vi "输入数据解析.vi"(0 "单个参数补充":dbl, 1 "从板号":dbl=1.0, 2 "主板二维码":string="BNET01", 3 "从板二维码":string="BNET01", 5 "主板引用":refnum<vi>, 7 "从板引用":refnum<vi>, 9 "主板选项":string="三级故障阀值", 11 "枚举":enum16{"主板", "从板"}(ring), 12 "快换":bool caption="快换写入") -> (4 "输出数组":dbl[][](array[numeric]), 6 "数组长度":dbl[](array[numeric]), 8 "循环次数":i32, 10 "命令":u32, 14 "名称":string[](array[string]), 15 "命令序号":u32[](array[numeric]))   [LabVIEW 2013] (continued)
                  disable-tunnel: [w17687 w17691] -> w17683
                  disable-tunnel: w17681 -> [w17686 _]
                  frame Disabled {
                    n6929 = Unbundle By Name(w17686) -> ("电压过高"=w17685:dbl)
                    n6930 = call "输入分辨率计算-EV05.vi"("1字节?"=FALSE, "数值"=w17685, "分辨率"=0.1) -> ("低字节"=w17687:dbl, "高字节1"=w17688:dbl)  [unwired: 2 in, 5 out]
                  }
                  frame Enabled {
                    w17691 = 255 ("高字节1")
                  }
                }
                n6931 = Build Array(w17684, w17683) -> (w17682:i32[])
              }
              frame 1 {
                # "电压过低"
                n6932 = disable-structure shown="启用" {
                  disable-tunnel: [w17699 w17702] -> w17695
                  disable-tunnel: [w17698 w17702] -> w17694
                  disable-tunnel: w17692 -> [w17697 _]
                  frame Disabled {
                    n6933 = Unbundle By Name(w17697) -> ("电压过低"=w17696:dbl)
                    n6934 = call "输入分辨率计算-EV05.vi"("1字节?"=FALSE, "数值"=w17696, "分辨率"=0.1) -> ("低字节"=w17698:dbl, "高字节1"=w17699:dbl)  [unwired: 2 in, 5 out]
                  }
                  frame Enabled {
                    w17702 = 255 ("高字节1")
                  }
                }
                n6935 = Build Array(w17695, w17694) -> (w17693:i32[])
              }
              frame 2 {
                # "电压不均衡"
                n6936 = disable-structure shown="启用" {
                  disable-tunnel: [w17710 w17713] -> w17706
                  disable-tunnel: [w17709 w17713] -> w17705
                  disable-tunnel: w17703 -> [w17708 _]
                  frame Disabled {
                    n6937 = Unbundle By Name(w17708) -> ("电压不均衡(V)"=w17707:dbl)
                    n6938 = call "输入分辨率计算-EV05.vi"("1字节?"=FALSE, "数值"=w17707, "分辨率"=0.1) -> ("低字节"=w17709:dbl, "高字节1"=w17710:dbl)  [unwired: 2 in, 5 out]
                  }
                  frame Enabled {
                    w17713 = 255 ("高字节1")
                  }
                }
                n6939 = Build Array(w17706, w17705) -> (w17704:i32[])
              }
              frame 3 {
                # "温度过高"
                n6940 = disable-structure shown="启用" {
                  disable-tunnel: [w17720 255 ("高字节1")] -> w17716
                  disable-tunnel: w17714 -> [w17718 _]
                  frame Enabled {
                    n6941 = Unbundle By Name(w17718) -> ("温度过高"=w17717:dbl)
                    n6942 = call "输入分辨率计算-EV05.vi"("1字节?"=TRUE, "数值"=w17717, "偏移量"=-40.0, "分辨率"=1.0) -> ("高字节1"=w17720:dbl)  [unwired: 1 in, 6 out]
                  }
                  frame Disabled {
                  }
                }
                n6943 = Build Array(w17716) -> (w17715:dbl[])
              }
              frame 4 {
                # "温度过低"
                n6944 = disable-structure shown="启用" {
                  disable-tunnel: [w17730 255 ("高字节1")] -> w17726
                  disable-tunnel: w17724 -> [w17728 _]
                  frame Disabled {
                    n6945 = Unbundle By Name(w17728) -> ("温度过低"=w17727:dbl)
                    n6946 = call "输入分辨率计算-EV05.vi"("1字节?"=TRUE, "数值"=w17727, "偏移量"=-40.0, "分辨率"=1.0) -> ("高字节1"=w17730:dbl)  [unwired: 1 in, 6 out]
                  }
                  frame Enabled {
                  }
                }
                n6947 = Build Array(w17726) -> (w17725:i32[])
              }
              frame 5 {
                # "温度不均衡"
                n6948 = disable-structure shown="启用" {
                  disable-tunnel: [w17739 255 ("高字节1")] -> w17736
                  disable-tunnel: w17734 -> [w17738 _]
                  frame Disabled {
                    n6949 = Unbundle By Name(w17738) -> ("温度不均衡"=w17737:dbl)
                    n6950 = call "输入分辨率计算-EV05.vi"("1字节?"=TRUE, "数值"=w17737, "分辨率"=1.0) -> ("高字节1"=w17739:dbl)  [unwired: 2 in, 6 out]
                  }
                  frame Enabled {
                  }
                }
                n6951 = Build Array(w17736) -> (w17735:i32[])
              }
              frame 6 {
                # "SOC过低"
                n6952 = disable-structure shown="启用" {
                  disable-tunnel: w17745 -> [w17762 _]
                  disable-tunnel: [w17748 w17765] -> w17744
                  disable-tunnel: [w17747 w17765] -> w17743
                  frame Disabled {
                    n6953 = Unbundle By Name(w17762) -> ("SOC过低"=w17761:dbl)
                    n6954 = call "输入分辨率计算-EV05.vi"("1字节?"=FALSE, "数值"=w17761, "分辨率"=0.1) -> ("低字节"=w17750:dbl, "高字节1"=w17751:dbl)  [unwired: 2 in, 5 out]
                    n6955 = call "二进制解析-8.6.vi"("索引"=4, "数值"=0) -> ("低位子数组"=w17754:i32[])  [unwired: 3 out]
                    n6956 = call "二进制解析-8.6.vi"("索引"=4, "数值"=w17751) -> ("低位子数组"=w17757:i32[])  [unwired: 3 out]
                    n6957 = call "二进制解析-8.6.vi"("索引"=4, "数值"=w17750) -> ("低位子数组"=w17755:i32[], "高位子数组"=w17756:i32[])  [unwired: 2 out]
                    n6958 = Insert Into Array(array=w17757, new element=w17756) -> (w17759:i32[])  [unwired: 1 in]
                    n6959 = Insert Into Array(array=w17755, new element=w17754) -> (w17753:i32[])  [unwired: 1 in]
                    n6960 = call "数值二进制转十进制-8.6.vi"("子数组"=w17753) -> ("十进制数值"=w17748:i32)  [unwired: 4 out]
                    n6961 = call "数值二进制转十进制-8.6.vi"("子数组"=w17759) -> ("十进制数值"=w17747:i32)  [unwired: 4 out]
                  }
                  frame Enabled {
                    w17765 = 255 ("高字节1")
                  }
                }
                n6962 = Build Array(w17743, w17744) -> (w17746:i32[])
              }
            }
            n6963 = Insert Into Array(array=w17677, new element=w17676) -> (w17678:dbl[])  [unwired: 1 in]
          }
          n6964 = Build Array(w17671) -> (w17670:dbl[][])
        }
        frame "温度过高(3)" {
          n6965 = Unbundle By Name(w17770) -> ("三级故障(从板)"=w17771:refnum<vi>)
          n6966 = property class="Clust (严格)"(reference=w17771) -> ("Value"=w17769:T8)  [unwired: 1 in, 2 out]
          n6967 = for {
            N: 7 -> [_]
            tunnel: w17769 -> [w17781]
            shift-right: [w17780] -> w17773
            shift-left: dbl[] [] -> [w17779]
            i -> [w17782]
            n6968 = case shown="3" w17782 {
              tunnel: w17781 -> [w17783 w17794 w17805 w17816 w17826 w17836 w17847]
              tunnel: [w17784 w17795 w17806 w17817 w17827 w17837 w17848] -> w17778
              frame 0, Default {
                # "电压过高"
                n6969 = disable-structure shown="启用" {
                  disable-tunnel: [w17790 w17793] -> w17786
                  disable-tunnel: [w17789 w17793] -> w17785
                  disable-tunnel: w17783 -> [w17788 _]
                  frame Disabled {
                    n6970 = Unbundle By Name(w17788) -> ("电压过高"=w17787:dbl)
                    n6971 = call "输入分辨率计算-EV05.vi"("1字节?"=FALSE, "数值"=w17787, "分辨率"=0.1) -> ("低字节"=w17789:dbl, "高字节1"=w17790:dbl)  [unwired: 2 in, 5 out]
                  }
                  frame Enabled {
                    w17793 = 255 ("高字节1")
                  }
                }
                n6972 = Build Array(w17786, w17785) -> (w17784:i32[])
              }
              frame 1 {
                # "电压过低"
                n6973 = disable-structure shown="启用" {
                  disable-tunnel: [w17801 w17804] -> w17797
                  disable-tunnel: [w17800 w17804] -> w17796
                  disable-tunnel: w17794 -> [w17799 _]
                  frame Disabled {
                    n6974 = Unbundle By Name(w17799) -> ("电压过低"=w17798:dbl)
                    n6975 = call "输入分辨率计算-EV05.vi"("1字节?"=FALSE, "数值"=w17798, "分辨率"=0.1) -> ("低字节"=w17800:dbl, "高字节1"=w17801:dbl)  [unwired: 2 in, 5 out]
                  }
                  frame Enabled {
                    w17804 = 255 ("高字节1")
                  }
                }
                n6976 = Build Array(w17797, w17796) -> (w17795:i32[])
              }
              frame 2 {
                # "电压不均衡"
                n6977 = disable-structure shown="启用" {
                  disable-tunnel: [w17812 w17815] -> w17808
                  disable-tunnel: [w17811 w17815] -> w17807
                  disable-tunnel: w17805 -> [w17810 _]
                  frame Disabled {
                    n6978 = Unbundle By Name(w17810) -> ("电压不均衡(V)"=w17809:dbl)
                    n6979 = call "输入分辨率计算-EV05.vi"("1字节?"=FALSE, "数值"=w17809, "分辨率"=0.1) -> ("低字节"=w17811:dbl, "高字节1"=w17812:dbl)  [unwired: 2 in, 5 out]
                  }
                  frame Enabled {
                    w17815 = 255 ("高字节1")
                  }
                }
                n6980 = Build Array(w17808, w17807) -> (w17806:i32[])
              }
              frame 3 {
                # "温度过高"
                n6981 = disable-structure shown="启用" {
                  disable-tunnel: [w17822 255 ("高字节1")] -> w17818
                  disable-tunnel: w17816 -> [w17820 _]
                  frame Enabled {
                    n6982 = Unbundle By Name(w17820) -> ("温度过高"=w17819:dbl)
                    n6983 = call "输入分辨率计算-EV05.vi"("1字节?"=TRUE, "数值"=w17819, "偏移量"=-40.0, "分辨率"=1.0) -> ("高字节1"=w17822:dbl)  [unwired: 1 in, 6 out]
                  }
                  frame Disabled {
                  }
                }
                n6984 = Build Array(w17818) -> (w17817:dbl[])
              }
              frame 4 {
                # "温度过低"
                n6985 = disable-structure shown="启用" {
                  disable-tunnel: [w17832 255 ("高字节1")] -> w17828
                  disable-tunnel: w17826 -> [w17830 _]
                  frame Disabled {
                    n6986 = Unbundle By Name(w17830) -> ("温度过低"=w17829:dbl)
                    n6987 = call "输入分辨率计算-EV05.vi"("1字节?"=TRUE, "数值"=w17829, "偏移量"=-40.0, "分辨率"=1.0) -> ("高字节1"=w17832:dbl)  [unwired: 1 in, 6 out]
                  }
                  frame Enabled {
                  }
                }
                n6988 = Build Array(w17828) -> (w17827:i32[])
              }
              frame 5 {
                # "温度不均衡"
                n6989 = disable-structure shown="启用" {
                  disable-tunnel: [w17841 255 ("高字节1")] -> w17838
                  disable-tunnel: w17836 -> [w17840 _]
                  frame Disabled {
                    n6990 = Unbundle By Name(w17840) -> ("温度不均衡"=w17839:dbl)
                    n6991 = call "输入分辨率计算-EV05.vi"("1字节?"=TRUE, "数值"=w17839, "分辨率"=1.0) -> ("高字节1"=w17841:dbl)  [unwired: 2 in, 6 out]
                  }
                  frame Enabled {
                  }
                }
                n6992 = Build Array(w17838) -> (w17837:i32[])
              }
              frame 6 {
                # "SOC过低"
                n6993 = disable-structure shown="启用" {
                  disable-tunnel: w17847 -> [w17864 _]
                  disable-tunnel: [w17850 w17867] -> w17846
                  disable-tunnel: [w17849 w17867] -> w17845
                  frame Disabled {
                    n6994 = Unbundle By Name(w17864) -> ("SOC过低"=w17863:dbl)
                    n6995 = call "输入分辨率计算-EV05.vi"("1字节?"=FALSE, "数值"=w17863, "分辨率"=0.1) -> ("低字节"=w17852:dbl, "高字节1"=w17853:dbl)  [unwired: 2 in, 5 out]
                    n6996 = call "二进制解析-8.6.vi"("索引"=4, "数值"=0) -> ("低位子数组"=w17856:i32[])  [unwired: 3 out]
                    n6997 = call "二进制解析-8.6.vi"("索引"=4, "数值"=w17853) -> ("低位子数组"=w17859:i32[])  [unwired: 3 out]
                    n6998 = call "二进制解析-8.6.vi"("索引"=4, "数值"=w17852) -> ("低位子数组"=w17857:i32[], "高位子数组"=w17858:i32[])  [unwired: 2 out]
                    n6999 = Insert Into Array(array=w17859, new element=w17858) -> (w17861:i32[])  [unwired: 1 in]
                    n7000 = Insert Into Array(array=w17857, new element=w17856) -> (w17855:i32[])  [unwired: 1 in]
                    n7001 = call "数值二进制转十进制-8.6.vi"("子数组"=w17855) -> ("十进制数值"=w17850:i32)  [unwired: 4 out]
                    n7002 = call "数值二进制转十进制-8.6.vi"("子数组"=w17861) -> ("十进制数值"=w17849:i32)  [unwired: 4 out]
                  }
                  frame Enabled {
                    w17867 = 255 ("高字节1")
                  }
                }
                n7003 = Build Array(w17845, w17846) -> (w17848:i32[])
              }
            }
            n7004 = Insert Into Array(array=w17779, new element=w17778) -> (w17780:dbl[])  [unwired: 1 in]
          }
          n7005 = Build Array(w17773) -> (w17772:dbl[][])
        }
        frame "温度过低" {
          n7006 = Unbundle By Name(w17872) -> ("一级故障(从板)"=w17873:refnum<vi>)
          n7007 = property class="Clust (严格)"(reference=w17873) -> ("Value"=w17871:T8)  [unwired: 1 in, 2 out]
          n7008 = for {
            N: 7 -> [_]
            tunnel: w17871 -> [w17883]
            shift-right: [w17882] -> w17875
            shift-left: dbl[] [] -> [w17881]
            i -> [w17884]
            n7009 = case shown="4" w17884 {
              tunnel: w17883 -> [w17885 w17896 w17907 w17918 w17928 w17938 w17949]
              tunnel: [w17886 w17897 w17908 w17919 w17929 w17939 w17950] -> w17880
              frame 0, Default {
                # "电压过高"
                n7010 = disable-structure shown="启用" {
                  disable-tunnel: [w17892 w17895] -> w17888
                  disable-tunnel: [w17891 w17895] -> w17887
                  disable-tunnel: w17885 -> [w17890 _]
                  frame Disabled {
                    n7011 = Unbundle By Name(w17890) -> ("电压过高"=w17889:dbl)
                    n7012 = call "输入分辨率计算-EV05.vi"("1字节?"=FALSE, "数值"=w17889, "分辨率"=0.1) -> ("低字节"=w17891:dbl, "高字节1"=w17892:dbl)  [unwired: 2 in, 5 out]
                  }
                  frame Enabled {
                    w17895 = 255 ("高字节1")
                  }
                }
                n7013 = Build Array(w17888, w17887) -> (w17886:i32[])
              }
              frame 1 {
                # "电压过低"
                n7014 = disable-structure shown="启用" {
                  disable-tunnel: [w17903 w17906] -> w17899
                  disable-tunnel: [w17902 w17906] -> w17898
                  disable-tunnel: w17896 -> [w17901 _]
                  frame Disabled {
                    n7015 = Unbundle By Name(w17901) -> ("电压过低"=w17900:dbl)
                    n7016 = call "输入分辨率计算-EV05.vi"("1字节?"=FALSE, "数值"=w17900, "分辨率"=0.1) -> ("低字节"=w17902:dbl, "高字节1"=w17903:dbl)  [unwired: 2 in, 5 out]
                  }
                  frame Enabled {
                    w17906 = 255 ("高字节1")
                  }
                }
                n7017 = Build Array(w17899, w17898) -> (w17897:i32[])
              }
              frame 2 {
                # "电压不均衡"
                n7018 = disable-structure shown="启用" {
                  disable-tunnel: [w17914 w17917] -> w17910
                  disable-tunnel: [w17913 w17917] -> w17909
                  disable-tunnel: w17907 -> [w17912 _]
                  frame Disabled {
                    n7019 = Unbundle By Name(w17912) -> ("电压不均衡(V)"=w17911:dbl)
                    n7020 = call "输入分辨率计算-EV05.vi"("1字节?"=FALSE, "数值"=w17911, "分辨率"=0.1) -> ("低字节"=w17913:dbl, "高字节1"=w17914:dbl)  [unwired: 2 in, 5 out]
                  }
                  frame Enabled {
                    w17917 = 255 ("高字节1")
                  }
                }
                n7021 = Build Array(w17910, w17909) -> (w17908:i32[])
              }
              frame 3 {
                # "温度过高"
                n7022 = disable-structure shown="启用" {
                  disable-tunnel: [w17924 255 ("高字节1")] -> w17920
                  disable-tunnel: w17918 -> [w17922 _]
                  frame Disabled {
                    n7023 = Unbundle By Name(w17922) -> ("温度过高"=w17921:dbl)
                    n7024 = call "输入分辨率计算-EV05.vi"("1字节?"=TRUE, "数值"=w17921, "偏移量"=-40.0, "分辨率"=1.0) -> ("高字节1"=w17924:dbl)  [unwired: 1 in, 6 out]
                  }
                  frame Enabled {
                  }
                }
                n7025 = Build Array(w17920) -> (w17919:i32[])
              }
              frame 4 {
                # "温度过低"
                n7026 = disable-structure shown="启用" {
                  disable-tunnel: [w17934 255 ("高字节1")] -> w17930
                  disable-tunnel: w17928 -> [w17932 _]
                  frame Enabled {
                    n7027 = Unbundle By Name(w17932) -> ("温度过低"=w17931:dbl)
                    n7028 = call "输入分辨率计算-EV05.vi"("1字节?"=TRUE, "数值"=w17931, "偏移量"=-40.0, "分辨率"=1.0) -> ("高字节1"=w17934:dbl)  [unwired: 1 in, 6 out]
                  }
                  frame Disabled {
                  }
                }
                n7029 = Build Array(w17930) -> (w17929:dbl[])
              }
              frame 5 {
                # "温度不均衡"
                n7030 = disable-structure shown="启用" {
                  disable-tunnel: [w17943 255 ("高字节1")] -> w17940
                  disable-tunnel: w17938 -> [w17942 _]
                  frame Disabled {
                    n7031 = Unbundle By Name(w17942) -> ("温度不均衡"=w17941:dbl)
                    n7032 = call "输入分辨率计算-EV05.vi"("1字节?"=TRUE, "数值"=w17941, "分辨率"=1.0) -> ("高字节1"=w17943:dbl)  [unwired: 2 in, 6 out]
                  }
                  frame Enabled {
                  }
                }
                n7033 = Build Array(w17940) -> (w17939:i32[])
              }
              frame 6 {
                # "SOC过低"
                n7034 = disable-structure shown="启用" {
                  disable-tunnel: w17949 -> [w17966 _]
                  disable-tunnel: [w17952 w17969] -> w17948
                  disable-tunnel: [w17951 w17969] -> w17947
                  frame Disabled {
                    n7035 = Unbundle By Name(w17966) -> ("SOC过低"=w17965:dbl)
                    n7036 = call "输入分辨率计算-EV05.vi"("1字节?"=FALSE, "数值"=w17965, "分辨率"=0.1) -> ("低字节"=w17954:dbl, "高字节1"=w17955:dbl)  [unwired: 2 in, 5 out]
                    n7037 = call "二进制解析-8.6.vi"("索引"=4, "数值"=0) -> ("低位子数组"=w17958:i32[])  [unwired: 3 out]
                    n7038 = call "二进制解析-8.6.vi"("索引"=4, "数值"=w17955) -> ("低位子数组"=w17961:i32[])  [unwired: 3 out]
                    n7039 = call "二进制解析-8.6.vi"("索引"=4, "数值"=w17954) -> ("低位子数组"=w17959:i32[], "高位子数组"=w17960:i32[])  [unwired: 2 out]
                    n7040 = Insert Into Array(array=w17961, new element=w17960) -> (w17963:i32[])  [unwired: 1 in]
                    n7041 = Insert Into Array(array=w17959, new element=w17958) -> (w17957:i32[])  [unwired: 1 in]
                    n7042 = call "数值二进制转十进制-8.6.vi"("子数组"=w17957) -> ("十进制数值"=w17952:i32)  [unwired: 4 out]
                    n7043 = call "数值二进制转十进制-8.6.vi"("子数组"=w17963) -> ("十进制数值"=w17951:i32)  [unwired: 4 out]
                  }
                  frame Enabled {
                    w17969 = 255 ("高字节1")
                  }
                }
                n7044 = Build Array(w17947, w17948) -> (w17950:i32[])
              }
            }
            n7045 = Insert Into Array(array=w17881, new element=w17880) -> (w17882:dbl[])  [unwired: 1 in]
          }
          n7046 = Build Array(w17875) -> (w17874:dbl[][])
        }
        frame "温度过低(2)" {
          n7047 = Unbundle By Name(w17974) -> ("二级故障(从板)"=w17975:refnum<vi>)
          n7048 = property class="Clust (严格)"(reference=w17975) -> ("Value"=w17973:T8)  [unwired: 1 in, 2 out]
          n7049 = for {
            N: 7 -> [_]
            tunnel: w17973 -> [w17985]
            shift-right: [w17984] -> w17977
            shift-left: dbl[] [] -> [w17983]
            i -> [w17986]
            n7050 = case shown="4" w17986 {
              tunnel: w17985 -> [w17987 w17998 w18009 w18020 w18030 w18040 w18051]
              tunnel: [w17988 w17999 w18010 w18021 w18031 w18041 w18052] -> w17982
              frame 0, Default {
                # "电压过高"
                n7051 = disable-structure shown="启用" {
                  disable-tunnel: [w17994 w17997] -> w17990
                  disable-tunnel: [w17993 w17997] -> w17989
                  disable-tunnel: w17987 -> [w17992 _]
                  frame Disabled {
                    n7052 = Unbundle By Name(w17992) -> ("电压过高"=w17991:dbl)
                    n7053 = call "输入分辨率计算-EV05.vi"("1字节?"=FALSE, "数值"=w17991, "分辨率"=0.1) -> ("低字节"=w17993:dbl, "高字节1"=w17994:dbl)  [unwired: 2 in, 5 out]
                  }
                  frame Enabled {
                    w17997 = 255 ("高字节1")
                  }
                }
                n7054 = Build Array(w17990, w17989) -> (w17988:i32[])
              }
              frame 1 {
                # "电压过低"
                n7055 = disable-structure shown="启用" {
                  disable-tunnel: [w18005 w18008] -> w18001
                  disable-tunnel: [w18004 w18008] -> w18000
                  disable-tunnel: w17998 -> [w18003 _]
                  frame Disabled {
                    n7056 = Unbundle By Name(w18003) -> ("电压过低"=w18002:dbl)
                    n7057 = call "输入分辨率计算-EV05.vi"("1字节?"=FALSE, "数值"=w18002, "分辨率"=0.1) -> ("低字节"=w18004:dbl, "高字节1"=w18005:dbl)  [unwired: 2 in, 5 out]
                  }
                  frame Enabled {
                    w18008 = 255 ("高字节1")
                  }
                }
                n7058 = Build Array(w18001, w18000) -> (w17999:i32[])
              }
              frame 2 {
                # "电压不均衡"
                n7059 = disable-structure shown="启用" {
                  disable-tunnel: [w18016 w18019] -> w18012
                  disable-tunnel: [w18015 w18019] -> w18011
                  disable-tunnel: w18009 -> [w18014 _]
                  frame Disabled {
                    n7060 = Unbundle By Name(w18014) -> ("电压不均衡(V)"=w18013:dbl)
                    n7061 = call "输入分辨率计算-EV05.vi"("1字节?"=FALSE, "数值"=w18013, "分辨率"=0.1) -> ("低字节"=w18015:dbl, "高字节1"=w18016:dbl)  [unwired: 2 in, 5 out]
                  }
                  frame Enabled {
                    w18019 = 255 ("高字节1")
                  }
                }
                n7062 = Build Array(w18012, w18011) -> (w18010:i32[])
              }
              frame 3 {
                # "温度过高"
                n7063 = disable-structure shown="启用" {
                  disable-tunnel: [w18026 255 ("高字节1")] -> w18022
                  disable-tunnel: w18020 -> [w18024 _]
                  frame Disabled {
                    n7064 = Unbundle By Name(w18024) -> ("温度过高"=w18023:dbl)
                    n7065 = call "输入分辨率计算-EV05.vi"("1字节?"=TRUE, "数值"=w18023, "偏移量"=-40.0, "分辨率"=1.0) -> ("高字节1"=w18026:dbl)  [unwired: 1 in, 6 out]
                  }
                  frame Enabled {
                  }
                }
                n7066 = Build Array(w18022) -> (w18021:i32[])
              }
              frame 4 {
                # "温度过低"
                n7067 = disable-structure shown="启用" {
                  disable-tunnel: [w18036 255 ("高字节1")] -> w18032
                  disable-tunnel: w18030 -> [w18034 _]
                  frame Enabled {
                    n7068 = Unbundle By Name(w18034) -> ("温度过低"=w18033:dbl)
                    n7069 = call "输入分辨率计算-EV05.vi"("1字节?"=TRUE, "数值"=w18033, "偏移量"=-40.0, "分辨率"=1.0) -> ("高字节1"=w18036:dbl)  [unwired: 1 in, 6 out]
                  }
                  frame Disabled {
                  }
                }
                n7070 = Build Array(w18032) -> (w18031:dbl[])
              }
              frame 5 {
                # "温度不均衡"
                n7071 = disable-structure shown="启用" {
                  disable-tunnel: [w18045 255 ("高字节1")] -> w18042
                  disable-tunnel: w18040 -> [w18044 _]
                  frame Disabled {
                    n7072 = Unbundle By Name(w18044) -> ("温度不均衡"=w18043:dbl)
                    n7073 = call "输入分辨率计算-EV05.vi"("1字节?"=TRUE, "数值"=w18043, "分辨率"=1.0) -> ("高字节1"=w18045:dbl)  [unwired: 2 in, 6 out]
                  }
                  frame Enabled {
                  }
                }
                n7074 = Build Array(w18042) -> (w18041:i32[])
              }
              frame 6 {
                # "SOC过低"
                n7075 = disable-structure shown="启用" {
                  disable-tunnel: w18051 -> [w18068 _]
                  disable-tunnel: [w18054 w18071] -> w18050
                  disable-tunnel: [w18053 w18071] -> w18049
                  frame Disabled {
                    n7076 = Unbundle By Name(w18068) -> ("SOC过低"=w18067:dbl)
                    n7077 = call "输入分辨率计算-EV05.vi"("1字节?"=FALSE, "数值"=w18067, "分辨率"=0.1) -> ("低字节"=w18056:dbl, "高字节1"=w18057:dbl)  [unwired: 2 in, 5 out]
                    n7078 = call "二进制解析-8.6.vi"("索引"=4, "数值"=0) -> ("低位子数组"=w18060:i32[])  [unwired: 3 out]
                    n7079 = call "二进制解析-8.6.vi"("索引"=4, "数值"=w18057) -> ("低位子数组"=w18063:i32[])  [unwired: 3 out]
                    n7080 = call "二进制解析-8.6.vi"("索引"=4, "数值"=w18056) -> ("低位子数组"=w18061:i32[], "高位子数组"=w18062:i32[])  [unwired: 2 out]
                    n7081 = Insert Into Array(array=w18063, new element=w18062) -> (w18065:i32[])  [unwired: 1 in]
                    n7082 = Insert Into Array(array=w18061, new element=w18060) -> (w18059:i32[])  [unwired: 1 in]
                    n7083 = call "数值二进制转十进制-8.6.vi"("子数组"=w18059) -> ("十进制数值"=w18054:i32)  [unwired: 4 out]
                    n7084 = call "数值二进制转十进制-8.6.vi"("子数组"=w18065) -> ("十进制数值"=w18053:i32)  [unwired: 4 out]
                  }
                  frame Enabled {
                    w18071 = 255 ("高字节1")
                  }
                }
                n7085 = Build Array(w18049, w18050) -> (w18052:i32[])
              }
            }
            n7086 = Insert Into Array(array=w17983, new element=w17982) -> (w17984:dbl[])  [unwired: 1 in]
          }
          n7087 = Build Array(w17977) -> (w17976:dbl[][])
        }
        frame "温度过低(3)" {
          n7088 = Unbundle By Name(w18076) -> ("三级故障(从板)"=w18077:refnum<vi>)
          n7089 = property class="Clust (严格)"(reference=w18077) -> ("Value"=w18075:T8)  [unwired: 1 in, 2 out]
          n7090 = for {
            N: 7 -> [_]
            tunnel: w18075 -> [w18087]
            shift-right: [w18086] -> w18079
            shift-left: dbl[] [] -> [w18085]
            i -> [w18088]
            n7091 = case shown="4" w18088 {
              tunnel: w18087 -> [w18089 w18100 w18111 w18122 w18132 w18142 w18153]
              tunnel: [w18090 w18101 w18112 w18123 w18133 w18143 w18154] -> w18084
              frame 0, Default {
                # "电压过高"
                n7092 = disable-structure shown="启用" {
                  disable-tunnel: [w18096 w18099] -> w18092
                  disable-tunnel: [w18095 w18099] -> w18091
                  disable-tunnel: w18089 -> [w18094 _]
                  frame Disabled {
                    n7093 = Unbundle By Name(w18094) -> ("电压过高"=w18093:dbl)
                    n7094 = call "输入分辨率计算-EV05.vi"("1字节?"=FALSE, "数值"=w18093, "分辨率"=0.1) -> ("低字节"=w18095:dbl, "高字节1"=w18096:dbl)  [unwired: 2 in, 5 out]
                  }
                  frame Enabled {
                    w18099 = 255 ("高字节1")
                  }
                }
                n7095 = Build Array(w18092, w18091) -> (w18090:i32[])
              }
              frame 1 {
                # "电压过低"
                n7096 = disable-structure shown="启用" {
                  disable-tunnel: [w18107 w18110] -> w18103
                  disable-tunnel: [w18106 w18110] -> w18102
                  disable-tunnel: w18100 -> [w18105 _]
                  frame Disabled {
                    n7097 = Unbundle By Name(w18105) -> ("电压过低"=w18104:dbl)
                    n7098 = call "输入分辨率计算-EV05.vi"("1字节?"=FALSE, "数值"=w18104, "分辨率"=0.1) -> ("低字节"=w18106:dbl, "高字节1"=w18107:dbl)  [unwired: 2 in, 5 out]
                  }
                  frame Enabled {
                    w18110 = 255 ("高字节1")
                  }
                }
                n7099 = Build Array(w18103, w18102) -> (w18101:i32[])
              }
              frame 2 {
                # "电压不均衡"
                n7100 = disable-structure shown="启用" {
                  disable-tunnel: [w18118 w18121] -> w18114
                  disable-tunnel: [w18117 w18121] -> w18113
                  disable-tunnel: w18111 -> [w18116 _]
                  frame Disabled {
                    n7101 = Unbundle By Name(w18116) -> ("电压不均衡(V)"=w18115:dbl)
                    n7102 = call "输入分辨率计算-EV05.vi"("1字节?"=FALSE, "数值"=w18115, "分辨率"=0.1) -> ("低字节"=w18117:dbl, "高字节1"=w18118:dbl)  [unwired: 2 in, 5 out]
                  }
                  frame Enabled {
                    w18121 = 255 ("高字节1")
                  }
                }
                n7103 = Build Array(w18114, w18113) -> (w18112:i32[])
              }
              frame 3 {
                # "温度过高"
                n7104 = disable-structure shown="启用" {
                  disable-tunnel: [w18128 255 ("高字节1")] -> w18124
                  disable-tunnel: w18122 -> [w18126 _]
                  frame Disabled {
                    n7105 = Unbundle By Name(w18126) -> ("温度过高"=w18125:dbl)
                    n7106 = call "输入分辨率计算-EV05.vi"("1字节?"=TRUE, "数值"=w18125, "偏移量"=-40.0, "分辨率"=1.0) -> ("高字节1"=w18128:dbl)  [unwired: 1 in, 6 out]
                  }
                  frame Enabled {
                  }
                }
                n7107 = Build Array(w18124) -> (w18123:i32[])
              }
              frame 4 {
                # "温度过低"
                n7108 = disable-structure shown="启用" {
                  disable-tunnel: [w18138 255 ("高字节1")] -> w18134
                  disable-tunnel: w18132 -> [w18136 _]
                  frame Enabled {
                    n7109 = Unbundle By Name(w18136) -> ("温度过低"=w18135:dbl)
                    n7110 = call "输入分辨率计算-EV05.vi"("1字节?"=TRUE, "数值"=w18135, "偏移量"=-40.0, "分辨率"=1.0) -> ("高字节1"=w18138:dbl)  [unwired: 1 in, 6 out]
                  }
                  frame Disabled {
                  }
                }
                n7111 = Build Array(w18134) -> (w18133:dbl[])
              }
              frame 5 {
                # "温度不均衡"
                n7112 = disable-structure shown="启用" {
                  disable-tunnel: [w18147 255 ("高字节1")] -> w18144
                  disable-tunnel: w18142 -> [w18146 _]
                  frame Disabled {
                    n7113 = Unbundle By Name(w18146) -> ("温度不均衡"=w18145:dbl)
                    n7114 = call "输入分辨率计算-EV05.vi"("1字节?"=TRUE, "数值"=w18145, "分辨率"=1.0) -> ("高字节1"=w18147:dbl)  [unwired: 2 in, 6 out]
                  }
                  frame Enabled {
                  }
                }
                n7115 = Build Array(w18144) -> (w18143:i32[])
              }
              frame 6 {
                # "SOC过低"
                n7116 = disable-structure shown="启用" {
                  disable-tunnel: w18153 -> [w18170 _]
                  disable-tunnel: [w18156 w18173] -> w18152
                  disable-tunnel: [w18155 w18173] -> w18151
                  frame Disabled {
                    n7117 = Unbundle By Name(w18170) -> ("SOC过低"=w18169:dbl)
                    n7118 = call "输入分辨率计算-EV05.vi"("1字节?"=FALSE, "数值"=w18169, "分辨率"=0.1) -> ("低字节"=w18158:dbl, "高字节1"=w18159:dbl)  [unwired: 2 in, 5 out]
                    n7119 = call "二进制解析-8.6.vi"("索引"=4, "数值"=0) -> ("低位子数组"=w18162:i32[])  [unwired: 3 out]
                    n7120 = call "二进制解析-8.6.vi"("索引"=4, "数值"=w18159) -> ("低位子数组"=w18165:i32[])  [unwired: 3 out]
                    n7121 = call "二进制解析-8.6.vi"("索引"=4, "数值"=w18158) -> ("低位子数组"=w18163:i32[], "高位子数组"=w18164:i32[])  [unwired: 2 out]
                    n7122 = Insert Into Array(array=w18165, new element=w18164) -> (w18167:i32[])  [unwired: 1 in]
                    n7123 = Insert Into Array(array=w18163, new element=w18162) -> (w18161:i32[])  [unwired: 1 in]
                    n7124 = call "数值二进制转十进制-8.6.vi"("子数组"=w18161) -> ("十进制数值"=w18156:i32)  [unwired: 4 out]
                    n7125 = call "数值二进制转十进制-8.6.vi"("子数组"=w18167) -> ("十进制数值"=w18155:i32)  [unwired: 4 out]
                  }
                  frame Enabled {
                    w18173 = 255 ("高字节1")
                  }
                }
                n7126 = Build Array(w18151, w18152) -> (w18154:i32[])
              }
            }
            n7127 = Insert Into Array(array=w18085, new element=w18084) -> (w18086:dbl[])  [unwired: 1 in]
          }
          n7128 = Build Array(w18079) -> (w18078:dbl[][])
        }
        frame "温度不均衡" {
          n7129 = Unbundle By Name(w18178) -> ("一级故障(从板)"=w18179:refnum<vi>)
          n7130 = property class="Clust (严格)"(reference=w18179) -> ("Value"=w18177:T8)  [unwired: 1 in, 2 out]
          n7131 = for {
            N: 7 -> [_]
            tunnel: w18177 -> [w18189]
            shift-right: [w18188] -> w18181
            shift-left: dbl[] [] -> [w18187]
            i -> [w18190]
            n7132 = case shown="5" w18190 {
              tunnel: w18189 -> [w18191 w18202 w18213 w18224 w18234 w18244 w18255]
              tunnel: [w18192 w18203 w18214 w18225 w18235 w18245 w18256] -> w18186
              frame 0, Default {
                # "电压过高"
                n7133 = disable-structure shown="启用" {
                  disable-tunnel: [w18198 w18201] -> w18194
                  disable-tunnel: [w18197 w18201] -> w18193
                  disable-tunnel: w18191 -> [w18196 _]
                  frame Disabled {
                    n7134 = Unbundle By Name(w18196) -> ("电压过高"=w18195:dbl)
                    n7135 = call "输入分辨率计算-EV05.vi"("1字节?"=FALSE, "数值"=w18195, "分辨率"=0.1) -> ("低字节"=w18197:dbl, "高字节1"=w18198:dbl)  [unwired: 2 in, 5 out]
                  }
                  frame Enabled {
                    w18201 = 255 ("高字节1")
                  }
                }
                n7136 = Build Array(w18194, w18193) -> (w18192:i32[])
              }
              frame 1 {
                # "电压过低"
                n7137 = disable-structure shown="启用" {
                  disable-tunnel: [w18209 w18212] -> w18205
                  disable-tunnel: [w18208 w18212] -> w18204
                  disable-tunnel: w18202 -> [w18207 _]
                  frame Disabled {
                    n7138 = Unbundle By Name(w18207) -> ("电压过低"=w18206:dbl)
                    n7139 = call "输入分辨率计算-EV05.vi"("1字节?"=FALSE, "数值"=w18206, "分辨率"=0.1) -> ("低字节"=w18208:dbl, "高字节1"=w18209:dbl)  [unwired: 2 in, 5 out]
                  }
                  frame Enabled {
                    w18212 = 255 ("高字节1")
                  }
                }
                n7140 = Build Array(w18205, w18204) -> (w18203:i32[])
              }
              frame 2 {
                # "电压不均衡"
                n7141 = disable-structure shown="启用" {
                  disable-tunnel: [w18220 w18223] -> w18216
                  disable-tunnel: [w18219 w18223] -> w18215
                  disable-tunnel: w18213 -> [w18218 _]
                  frame Disabled {
                    n7142 = Unbundle By Name(w18218) -> ("电压不均衡(V)"=w18217:dbl)
                    n7143 = call "输入分辨率计算-EV05.vi"("1字节?"=FALSE, "数值"=w18217, "分辨率"=0.1) -> ("低字节"=w18219:dbl, "高字节1"=w18220:dbl)  [unwired: 2 in, 5 out]
                  }
                  frame Enabled {
                    w18223 = 255 ("高字节1")
                  }
                }
                n7144 = Build Array(w18216, w18215) -> (w18214:i32[])
              }
              frame 3 {
                # "温度过高"
                n7145 = disable-structure shown="启用" {
                  disable-tunnel: [w18230 255 ("高字节1")] -> w18226
                  disable-tunnel: w18224 -> [w18228 _]
                  frame Disabled {
                    n7146 = Unbundle By Name(w18228) -> ("温度过高"=w18227:dbl)
                    n7147 = call "输入分辨率计算-EV05.vi"("1字节?"=TRUE, "数值"=w18227, "偏移量"=-40.0, "分辨率"=1.0) -> ("高字节1"=w18230:dbl)  [unwired: 1 in, 6 out]
                  }
                  frame Enabled {
                  }
                }
                n7148 = Build Array(w18226) -> (w18225:i32[])
              }
              frame 4 {
                # "温度过低"
                n7149 = disable-structure shown="启用" {
                  disable-tunnel: [w18240 255 ("高字节1")] -> w18236
                  disable-tunnel: w18234 -> [w18238 _]
                  frame Disabled {
                    n7150 = Unbundle By Name(w18238) -> ("温度过低"=w18237:dbl)
                    n7151 = call "输入分辨率计算-EV05.vi"("1字节?"=TRUE, "数值"=w18237, "偏移量"=-40.0, "分辨率"=1.0) -> ("高字节1"=w18240:dbl)  [unwired: 1 in, 6 out]
                  }
                  frame Enabled {
                  }
                }
                n7152 = Build Array(w18236) -> (w18235:i32[])
              }
              frame 5 {
                # "温度不均衡"
                n7153 = disable-structure shown="启用" {
                  disable-tunnel: [w18249 255 ("高字节1")] -> w18246
                  disable-tunnel: w18244 -> [w18248 _]
                  frame Enabled {
                    n7154 = Unbundle By Name(w18248) -> ("温度不均衡"=w18247:dbl)
                    n7155 = call "输入分辨率计算-EV05.vi"("1字节?"=TRUE, "数值"=w18247, "分辨率"=1.0) -> ("高字节1"=w18249:dbl)  [unwired: 2 in, 6 out]
                  }
                  frame Disabled {
                  }
                }
                n7156 = Build Array(w18246) -> (w18245:dbl[])
              }
              frame 6 {
                # "SOC过低"
                n7157 = disable-structure shown="启用" {
                  disable-tunnel: w18255 -> [w18272 _]
                  disable-tunnel: [w18258 w18275] -> w18254
                  disable-tunnel: [w18257 w18275] -> w18253
                  frame Disabled {
                    n7158 = Unbundle By Name(w18272) -> ("SOC过低"=w18271:dbl)
                    n7159 = call "输入分辨率计算-EV05.vi"("1字节?"=FALSE, "数值"=w18271, "分辨率"=0.1) -> ("低字节"=w18260:dbl, "高字节1"=w18261:dbl)  [unwired: 2 in, 5 out]
                    n7160 = call "二进制解析-8.6.vi"("索引"=4, "数值"=0) -> ("低位子数组"=w18264:i32[])  [unwired: 3 out]
                    n7161 = call "二进制解析-8.6.vi"("索引"=4, "数值"=w18261) -> ("低位子数组"=w18267:i32[])  [unwired: 3 out]
                    n7162 = call "二进制解析-8.6.vi"("索引"=4, "数值"=w18260) -> ("低位子数组"=w18265:i32[], "高位子数组"=w18266:i32[])  [unwired: 2 out]
                    n7163 = Insert Into Array(array=w18267, new element=w18266) -> (w18269:i32[])  [unwired: 1 in]
                    n7164 = Insert Into Array(array=w18265, new element=w18264) -> (w18263:i32[])  [unwired: 1 in]
                    n7165 = call "数值二进制转十进制-8.6.vi"("子数组"=w18263) -> ("十进制数值"=w18258:i32)  [unwired: 4 out]
                    n7166 = call "数值二进制转十进制-8.6.vi"("子数组"=w18269) -> ("十进制数值"=w18257:i32)  [unwired: 4 out]
                  }
                  frame Enabled {
                    w18275 = 255 ("高字节1")
                  }
                }
                n7167 = Build Array(w18253, w18254) -> (w18256:i32[])
              }
            }
            n7168 = Insert Into Array(array=w18187, new element=w18186) -> (w18188:dbl[])  [unwired: 1 in]
          }
          n7169 = Build Array(w18181) -> (w18180:dbl[][])
        }
        frame "温度不均衡(2)" {
          n7170 = Unbundle By Name(w18280) -> ("二级故障(从板)"=w18281:refnum<vi>)
          n7171 = property class="Clust (严格)"(reference=w18281) -> ("Value"=w18279:T8)  [unwired: 1 in, 2 out]
          n7172 = for {
            N: 7 -> [_]
            tunnel: w18279 -> [w18291]
            shift-right: [w18290] -> w18283
            shift-left: dbl[] [] -> [w18289]
            i -> [w18292]
            n7173 = case shown="5" w18292 {
              tunnel: w18291 -> [w18293 w18304 w18315 w18326 w18336 w18346 w18357]
              tunnel: [w18294 w18305 w18316 w18327 w18337 w18347 w18358] -> w18288
              frame 0, Default {
                # "电压过高"
                n7174 = disable-structure shown="启用" {
                  disable-tunnel: [w18300 w18303] -> w18296
                  disable-tunnel: [w18299 w18303] -> w18295
                  disable-tunnel: w18293 -> [w18298 _]
                  frame Disabled {
                    n7175 = Unbundle By Name(w18298) -> ("电压过高"=w18297:dbl)
                    n7176 = call "输入分辨率计算-EV05.vi"("1字节?"=FALSE, "数值"=w18297, "分辨率"=0.1) -> ("低字节"=w18299:dbl, "高字节1"=w18300:dbl)  [unwired: 2 in, 5 out]
                  }
                  frame Enabled {
                    w18303 = 255 ("高字节1")
                  }
                }
                n7177 = Build Array(w18296, w18295) -> (w18294:i32[])
              }
              frame 1 {
                # "电压过低"
                n7178 = disable-structure shown="启用" {
                  disable-tunnel: [w18311 w18314] -> w18307
                  disable-tunnel: [w18310 w18314] -> w18306
                  disable-tunnel: w18304 -> [w18309 _]
                  frame Disabled {
                    n7179 = Unbundle By Name(w18309) -> ("电压过低"=w18308:dbl)
                    n7180 = call "输入分辨率计算-EV05.vi"("1字节?"=FALSE, "数值"=w18308, "分辨率"=0.1) -> ("低字节"=w18310:dbl, "高字节1"=w18311:dbl)  [unwired: 2 in, 5 out]
                  }
                  frame Enabled {
                    w18314 = 255 ("高字节1")
                  }
                }
                n7181 = Build Array(w18307, w18306) -> (w18305:i32[])
              }
              frame 2 {
                # "电压不均衡"
                n7182 = disable-structure shown="启用" {
                  disable-tunnel: [w18322 w18325] -> w18318
                  disable-tunnel: [w18321 w18325] -> w18317
                  disable-tunnel: w18315 -> [w18320 _]
                  frame Disabled {
                    n7183 = Unbundle By Name(w18320) -> ("电压不均衡(V)"=w18319:dbl)
                    n7184 = call "输入分辨率计算-EV05.vi"("1字节?"=FALSE, "数值"=w18319, "分辨率"=0.1) -> ("低字节"=w18321:dbl, "高字节1"=w18322:dbl)  [unwired: 2 in, 5 out]
                  }
                  frame Enabled {
                    w18325 = 255 ("高字节1")
                  }
                }
                n7185 = Build Array(w18318, w18317) -> (w18316:i32[])
              }
              frame 3 {
                # "温度过高"
                n7186 = disable-structure shown="启用" {
                  disable-tunnel: [w18332 255 ("高字节1")] -> w18328
                  disable-tunnel: w18326 -> [w18330 _]
                  frame Disabled {
                    n7187 = Unbundle By Name(w18330) -> ("温度过高"=w18329:dbl)
                    n7188 = call "输入分辨率计算-EV05.vi"("1字节?"=TRUE, "数值"=w18329, "偏移量"=-40.0, "分辨率"=1.0) -> ("高字节1"=w18332:dbl)  [unwired: 1 in, 6 out]
                  }
                  frame Enabled {
                  }
                }
                n7189 = Build Array(w18328) -> (w18327:i32[])
              }
              frame 4 {
                # "温度过低"
                n7190 = disable-structure shown="启用" {
                  disable-tunnel: [w18342 255 ("高字节1")] -> w18338
                  disable-tunnel: w18336 -> [w18340 _]
                  frame Disabled {
                    n7191 = Unbundle By Name(w18340) -> ("温度过低"=w18339:dbl)
                    n7192 = call "输入分辨率计算-EV05.vi"("1字节?"=TRUE, "数值"=w18339, "偏移量"=-40.0, "分辨率"=1.0) -> ("高字节1"=w18342:dbl)  [unwired: 1 in, 6 out]
                  }
                  frame Enabled {
                  }
                }
                n7193 = Build Array(w18338) -> (w18337:i32[])
              }
              frame 5 {
                # "温度不均衡"
                n7194 = disable-structure shown="启用" {
                  disable-tunnel: [w18351 255 ("高字节1")] -> w18348
                  disable-tunnel: w18346 -> [w18350 _]
                  frame Enabled {
                    n7195 = Unbundle By Name(w18350) -> ("温度不均衡"=w18349:dbl)
                    n7196 = call "输入分辨率计算-EV05.vi"("1字节?"=TRUE, "数值"=w18349, "分辨率"=1.0) -> ("高字节1"=w18351:dbl)  [unwired: 2 in, 6 out]
                  }
                  frame Disabled {
                  }
                }
                n7197 = Build Array(w18348) -> (w18347:dbl[])
              }
              frame 6 {
                # "SOC过低"
                n7198 = disable-structure shown="启用" {
                  disable-tunnel: w18357 -> [w18374 _]
                  disable-tunnel: [w18360 w18377] -> w18356
                  disable-tunnel: [w18359 w18377] -> w18355
                  frame Disabled {
                    n7199 = Unbundle By Name(w18374) -> ("SOC过低"=w18373:dbl)
                    n7200 = call "输入分辨率计算-EV05.vi"("1字节?"=FALSE, "数值"=w18373, "分辨率"=0.1) -> ("低字节"=w18362:dbl, "高字节1"=w18363:dbl)  [unwired: 2 in, 5 out]
                    n7201 = call "二进制解析-8.6.vi"("索引"=4, "数值"=0) -> ("低位子数组"=w18366:i32[])  [unwired: 3 out]
                    n7202 = call "二进制解析-8.6.vi"("索引"=4, "数值"=w18363) -> ("低位子数组"=w18369:i32[])  [unwired: 3 out]
                    n7203 = call "二进制解析-8.6.vi"("索引"=4, "数值"=w18362) -> ("低位子数组"=w18367:i32[], "高位子数组"=w18368:i32[])  [unwired: 2 out]
                    n7204 = Insert Into Array(array=w18369, new element=w18368) -> (w18371:i32[])  [unwired: 1 in]
                    n7205 = Insert Into Array(array=w18367, new element=w18366) -> (w18365:i32[])  [unwired: 1 in]
                    n7206 = call "数值二进制转十进制-8.6.vi"("子数组"=w18365) -> ("十进制数值"=w18360:i32)  [unwired: 4 out]
                    n7207 = call "数值二进制转十进制-8.6.vi"("子数组"=w18371) -> ("十进制数值"=w18359:i32)  [unwired: 4 out]
                  }
                  frame Enabled {
                    w18377 = 255 ("高字节1")
                  }
                }
                n7208 = Build Array(w18355, w18356) -> (w18358:i32[])
              }
            }
            n7209 = Insert Into Array(array=w18289, new element=w18288) -> (w18290:dbl[])  [unwired: 1 in]
          }
          n7210 = Build Array(w18283) -> (w18282:dbl[][])
        }
        frame "温度不均衡(3)" {
          n7211 = Unbundle By Name(w18382) -> ("三级故障(从板)"=w18383:refnum<vi>)
          n7212 = property class="Clust (严格)"(reference=w18383) -> ("Value"=w18381:T8)  [unwired: 1 in, 2 out]
          n7213 = for {
            N: 7 -> [_]
            tunnel: w18381 -> [w18393]
            shift-right: [w18392] -> w18385
            shift-left: dbl[] [] -> [w18391]
            i -> [w18394]
            n7214 = case shown="5" w18394 {
              tunnel: w18393 -> [w18395 w18406 w18417 w18428 w18438 w18448 w18459]
              tunnel: [w18396 w18407 w18418 w18429 w18439 w18449 w18460] -> w18390
              frame 0, Default {
                # "电压过高"
                n7215 = disable-structure shown="启用" {
                  disable-tunnel: [w18402 w18405] -> w18398
                  disable-tunnel: [w18401 w18405] -> w18397
                  disable-tunnel: w18395 -> [w18400 _]
                  frame Disabled {
                    n7216 = Unbundle By Name(w18400) -> ("电压过高"=w18399:dbl)
                    n7217 = call "输入分辨率计算-EV05.vi"("1字节?"=FALSE, "数值"=w18399, "分辨率"=0.1) -> ("低字节"=w18401:dbl, "高字节1"=w18402:dbl)  [unwired: 2 in, 5 out]
                  }
                  frame Enabled {
                    w18405 = 255 ("高字节1")
                  }
                }
                n7218 = Build Array(w18398, w18397) -> (w18396:i32[])
              }
              frame 1 {
                # "电压过低"
                n7219 = disable-structure shown="启用" {
                  disable-tunnel: [w18413 w18416] -> w18409
                  disable-tunnel: [w18412 w18416] -> w18408
                  disable-tunnel: w18406 -> [w18411 _]
                  frame Disabled {
                    n7220 = Unbundle By Name(w18411) -> ("电压过低"=w18410:dbl)
                    n7221 = call "输入分辨率计算-EV05.vi"("1字节?"=FALSE, "数值"=w18410, "分辨率"=0.1) -> ("低字节"=w18412:dbl, "高字节1"=w18413:dbl)  [unwired: 2 in, 5 out]
                  }
                  frame Enabled {
                    w18416 = 255 ("高字节1")
                  }
                }
                n7222 = Build Array(w18409, w18408) -> (w18407:i32[])
              }
              frame 2 {
                # "电压不均衡"
                n7223 = disable-structure shown="启用" {
                  disable-tunnel: [w18424 w18427] -> w18420
                  disable-tunnel: [w18423 w18427] -> w18419
                  disable-tunnel: w18417 -> [w18422 _]
                  frame Disabled {
                    n7224 = Unbundle By Name(w18422) -> ("电压不均衡(V)"=w18421:dbl)
                    n7225 = call "输入分辨率计算-EV05.vi"("1字节?"=FALSE, "数值"=w18421, "分辨率"=0.1) -> ("低字节"=w18423:dbl, "高字节1"=w18424:dbl)  [unwired: 2 in, 5 out]
                  }
                  frame Enabled {
                    w18427 = 255 ("高字节1")
                  }
                }
                n7226 = Build Array(w18420, w18419) -> (w18418:i32[])
              }
              frame 3 {
                # "温度过高"
                n7227 = disable-structure shown="启用" {
                  disable-tunnel: [w18434 255 ("高字节1")] -> w18430
                  disable-tunnel: w18428 -> [w18432 _]
                  frame Disabled {
                    n7228 = Unbundle By Name(w18432) -> ("温度过高"=w18431:dbl)
                    n7229 = call "输入分辨率计算-EV05.vi"("1字节?"=TRUE, "数值"=w18431, "偏移量"=-40.0, "分辨率"=1.0) -> ("高字节1"=w18434:dbl)  [unwired: 1 in, 6 out]
                  }
                  frame Enabled {
                  }
                }
                n7230 = Build Array(w18430) -> (w18429:i32[])
              }
              frame 4 {
                # "温度过低"
                n7231 = disable-structure shown="启用" {
                  disable-tunnel: [w18444 255 ("高字节1")] -> w18440
                  disable-tunnel: w18438 -> [w18442 _]
                  frame Disabled {
                    n7232 = Unbundle By Name(w18442) -> ("温度过低"=w18441:dbl)
                    n7233 = call "输入分辨率计算-EV05.vi"("1字节?"=TRUE, "数值"=w18441, "偏移量"=-40.0, "分辨率"=1.0) -> ("高字节1"=w18444:dbl)  [unwired: 1 in, 6 out]
                  }
                  frame Enabled {
                  }
                }
                n7234 = Build Array(w18440) -> (w18439:i32[])
              }
              frame 5 {
                # "温度不均衡"
                n7235 = disable-structure shown="启用" {
                  disable-tunnel: [w18453 255 ("高字节1")] -> w18450
                  disable-tunnel: w18448 -> [w18452 _]
                  frame Enabled {
                    n7236 = Unbundle By Name(w18452) -> ("温度不均衡"=w18451:dbl)
                    n7237 = call "输入分辨率计算-EV05.vi"("1字节?"=TRUE, "数值"=w18451, "分辨率"=1.0) -> ("高字节1"=w18453:dbl)  [unwired: 2 in, 6 out]
                  }
                  frame Disabled {
                  }
                }
                n7238 = Build Array(w18450) -> (w18449:dbl[])
              }
              frame 6 {
                # "SOC过低"
                n7239 = disable-structure shown="启用" {
                  disable-tunnel: w18459 -> [w18476 _]
                  disable-tunnel: [w18462 w18479] -> w18458
                  disable-tunnel: [w18461 w18479] -> w18457
                  frame Disabled {
                    n7240 = Unbundle By Name(w18476) -> ("SOC过低"=w18475:dbl)
                    n7241 = call "输入分辨率计算-EV05.vi"("1字节?"=FALSE, "数值"=w18475, "分辨率"=0.1) -> ("低字节"=w18464:dbl, "高字节1"=w18465:dbl)  [unwired: 2 in, 5 out]
                    n7242 = call "二进制解析-8.6.vi"("索引"=4, "数值"=0) -> ("低位子数组"=w18468:i32[])  [unwired: 3 out]
                    n7243 = call "二进制解析-8.6.vi"("索引"=4, "数值"=w18465) -> ("低位子数组"=w18471:i32[])  [unwired: 3 out]
                    n7244 = call "二进制解析-8.6.vi"("索引"=4, "数值"=w18464) -> ("低位子数组"=w18469:i32[], "高位子数组"=w18470:i32[])  [unwired: 2 out]
                    n7245 = Insert Into Array(array=w18471, new element=w18470) -> (w18473:i32[])  [unwired: 1 in]
                    n7246 = Insert Into Array(array=w18469, new element=w18468) -> (w18467:i32[])  [unwired: 1 in]
                    n7247 = call "数值二进制转十进制-8.6.vi"("子数组"=w18467) -> ("十进制数值"=w18462:i32)  [unwired: 4 out]
                    n7248 = call "数值二进制转十进制-8.6.vi"("子数组"=w18473) -> ("十进制数值"=w18461:i32)  [unwired: 4 out]
                  }
                  frame Enabled {
                    w18479 = 255 ("高字节1")
                  }
                }
                n7249 = Build Array(w18457, w18458) -> (w18460:i32[])
              }
            }
            n7250 = Insert Into Array(array=w18391, new element=w18390) -> (w18392:dbl[])  [unwired: 1 in]
          }
          n7251 = Build Array(w18385) -> (w18384:dbl[][])
        }
        frame "SOC过低" {
          n7252 = Unbundle By Name(w18484) -> ("一级故障(从板)"=w18485:refnum<vi>)
          n7253 = property class="Clust (严格)"(reference=w18485) -> ("Value"=w18483:T8)  [unwired: 1 in, 2 out]
          n7254 = for {
            N: 7 -> [_]
            tunnel: w18483 -> [w18495]
            shift-right: [w18494] -> w18487
            shift-left: dbl[] [] -> [w18493]
            i -> [w18496]
            n7255 = case shown="6" w18496 {
              tunnel: w18495 -> [w18497 w18508 w18519 w18530 w18540 w18550 w18561]
